vi "Destroy Front Panel Events.vi"(8 "error in (no error)":errorcluster, 11 "Splash Screen in":refnum<class "Splash Screen.lvclass">) -> (0 "error out":errorcluster, 3 "Splash Screen out":refnum<class "Splash Screen.lvclass">)   [LabVIEW 2015, in "Splash Screen.lvlib" / "Splash Screen.lvclass"]
uses:
  Splash Screen.lvclass
  UI Window/UI Window.lvclass
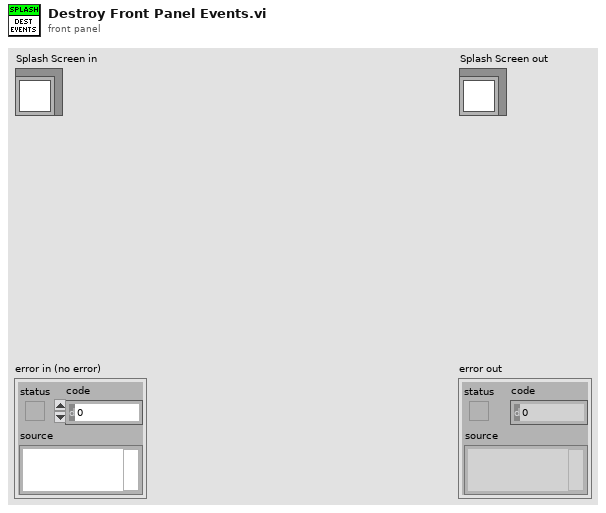
[diagram p1: front panel]
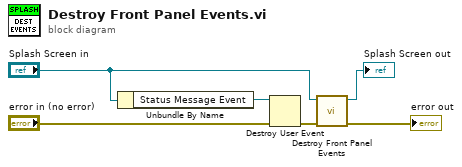
[diagram p0: block diagram]
diagram:
  n1 = Unbundle By Name("Splash Screen in") -> ("Status Message Event"=w4:refnum<user-event>)
  n2 = Destroy User Event(user event=w4, error in="error in (no error)") -> (error out=w1:errorcluster)
  n3 = call-parent "Destroy Front Panel Events.vi"("error in (no error)"=w1, "UI Window in"="Splash Screen in") -> ("error out"=→"error out":errorcluster, "UI Window out"=→"Splash Screen out":refnum<class "Splash Screen.lvclass">)  [unwired: 8 in]
